vi "Voltage - Continuous Input.vi"() -> ()   [LabVIEW 2012]
doc: "This example demonstrates how to continuously acquire buffered voltage measurements using a DAQmx device.\n\nFor instructions on how to connect your signals to the DAQ device, refer to your device documentation."
uses:
  <vilib>/DAQmx/read.llb/DAQmx Read (Analog 2D DBL NChan NSamp).vi
  <vilib>/DAQmx/create/channels.llb/DAQmx Create Channel (AI-Voltage-Basic).vi
  <vilib>/DAQmx/configure/timing.llb/DAQmx Timing (Sample Clock).vi
  <vilib>/DAQmx/miscellaneous.llb/DAQmx Fill In Error Info.vi
  <resource>/objmgr/daqmx.rc
panel:
  out "concatenated string":string
  out "Max Channels":i16
  in  "Over Sample factor":i16=1000
  out "data":dbl[][](array[numeric]) format="%.4f"
  out "Waveform Chart":dbl[][](graph)
  in  "Stop":bool
  in  "Sample Rate":dbl=1000.0
  in  "Sample Clock Source":tag="OnboardClock"
  in  "Terminal Configuration":i32(ring)=-1 items=["RSE"=10083, "Differential"=10106]
  in  "Max Voltage":dbl=5.0
  in  "Min Voltage":dbl=-5.0
  out "Actual Sample Rate":dbl=1000.0 format="%0.2f"
  # "Channel Settings"
  # "Acquired Data"
  # "Timing Settings"
  # "Logging Settings"
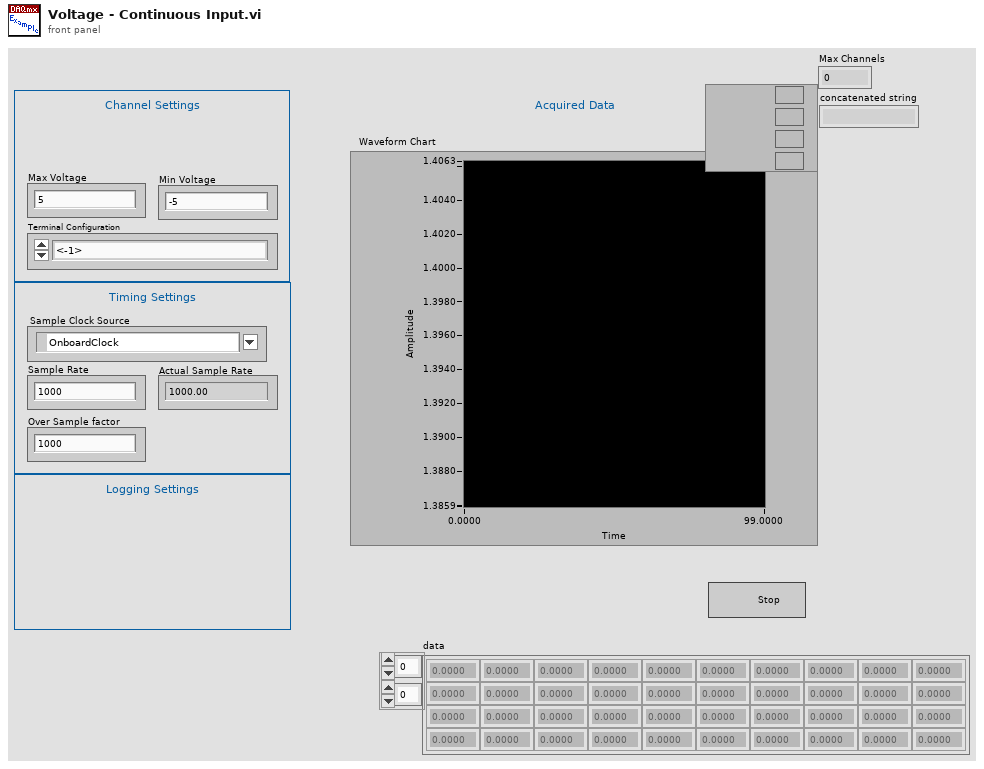
[diagram p1: front panel]
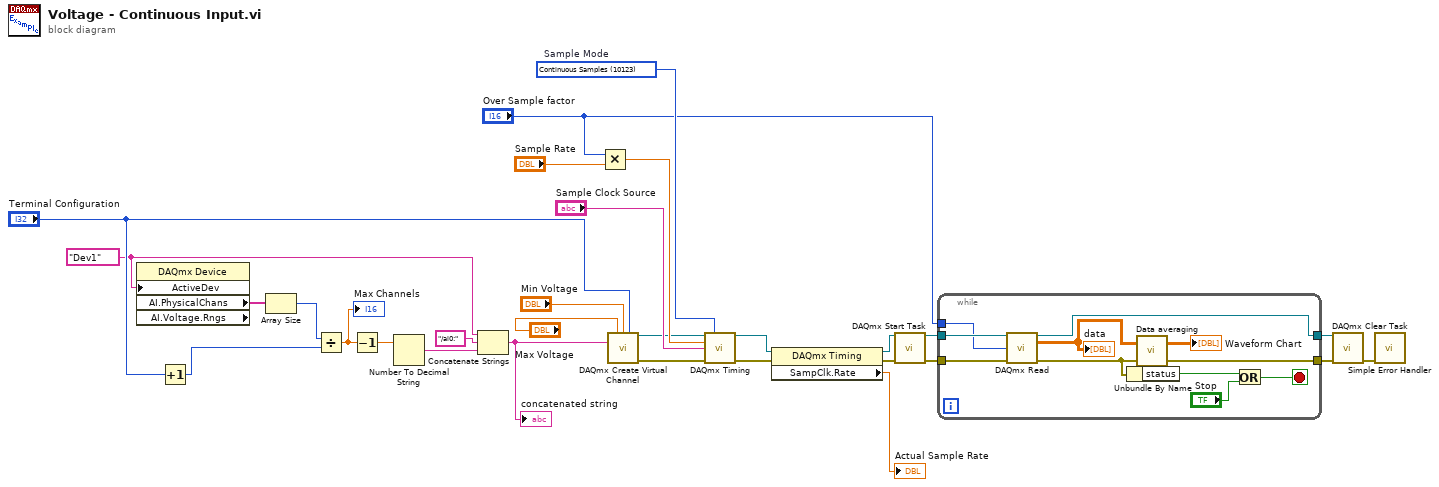
[diagram p0: block diagram]
diagram:
  w7 = tag "Dev1" ("device in")
  w27 = 10123 items=["Finite Samples"=10178, "Continuous Samples"=10123, "Hardware Timed Single Point"=12522]  # Sample Mode
  n1 = property class="DAQmx Device" props=["ActiveDev", "AI.PhysicalChans", "AI.Voltage.Rngs"]("ActiveDev"=w7) -> ("AI.PhysicalChans"=w9:tag[])  [unwired: 2 in, 3 out]
  n2 = Increment(x="Terminal Configuration") -> (x+1=w1:i32)
  n3 = Array Size(array=w9) -> (size(s)=w11:i32)
  n4 = Divide(x=w11, y=w1) -> (x/y=w5:dbl)
  "Max Channels" <- w5
  n5 = Decrement(x=w5) -> (x-1=w4:dbl)
  n6 = Number To Decimal String(number=w4) -> (decimal integer string=w3:string)  [unwired: 1 in]
  n7 = Concatenate Strings(w7, "/ai0:" ("string"), w3) -> (w2:string)
  "concatenated string" <- w2
  n8 = Multiply(x="Over Sample factor", y="Sample Rate") -> (x*y=w12:dbl)
  n9 = call-poly <vilib>:"DAQmx Create Virtual Channel.vi"("maximum value"="Max Voltage", "minimum value"="Min Voltage", "input terminal configuration"="Terminal Configuration", "physical channels"=w2) -> ("task out"=w10:refnum<k21>, "error out"=w26:errorcluster)  [unwired: 10 in]
  n10 = call-poly <vilib>:"DAQmx Timing.vi"("task/channels in"=w10, "sample mode"=w27, "rate"=w12, "source"="Sample Clock Source", "error in"=w26) -> ("task out"=w29:refnum<k21>, "error out"=w28:errorcluster)  [unwired: 9 in]
  n11 = property class="DAQmx Timing"(reference=w29, error in=w28) -> (reference out=w16:refnum<k21>, error out=w15:errorcluster, "SampClk.Rate"=→"Actual Sample Rate":dbl)
  n12 = call <vilib>:"DAQmx Start Task.vi"("task/channels in"=w16, "error in"=w15) -> ("task out"=w25:refnum<k21>, "error out"=w24:errorcluster)  [unwired: 12 in]
  n13 = while {
    tunnel: w25 -> [w39]
    tunnel: w24 -> [w38]
    tunnel: [w35] -> w22
    tunnel: [w36] -> w23
    tunnel: "Over Sample factor" -> [w30]
    stop <- w37 stop-if-true
    n14 = call-poly <vilib>:"DAQmx Read.vi"("task/channels in"=w39, "number of samples per channel"=w30, "error in"=w38) -> ("task out"=w36:refnum<k21>, "data"=w32:dbl[][], "error out"=w35:errorcluster)  [unwired: 10 in]
    "data" <- w32
    n15 = Unbundle By Name(w35) -> ("status"=w34:bool)
    n16 = call "Data averaging.vi"("data"=w32) -> ("Averaged data"=→"Waveform Chart":dbl[][])  [unwired: 2 in]
    n17 = Or(x=w34, y="Stop") -> (x .or. y?=w37:bool)
  }
  n18 = call <vilib>:"DAQmx Clear Task.vi"("task in"=w23, "error in"=w22) -> ("error out"=w21:errorcluster)  [unwired: 13 in]
  n19 = call <vilib>:"Simple Error Handler.vi"("error in (no error)"=w21) -> ()  [unwired: 4 in, 5 out]
